vi "Lidar.vi"() -> ()   [LabVIEW 2018]
uses:
  <vilib>/Tufts CEEO ROS for LabVIEW Software/ROS/Code/Console/Servers/ServerSubs/TopicDef.ctl
  <vilib>/Tufts CEEO ROS for LabVIEW Software/ROS/Code/SubVIs/_ROSDirection.ctl
  <vilib>/Utility/inputDevices.llb/keyboardAcquire.vi
  <vilib>/Utility/inputDevices.llb/closeKeyboard.vi
panel:
  out "keyType 3":T1(ring)
  in  "stop 2":bool
  out "new picture":picture
  out "msg out":string
  out "PoseStamped":T2
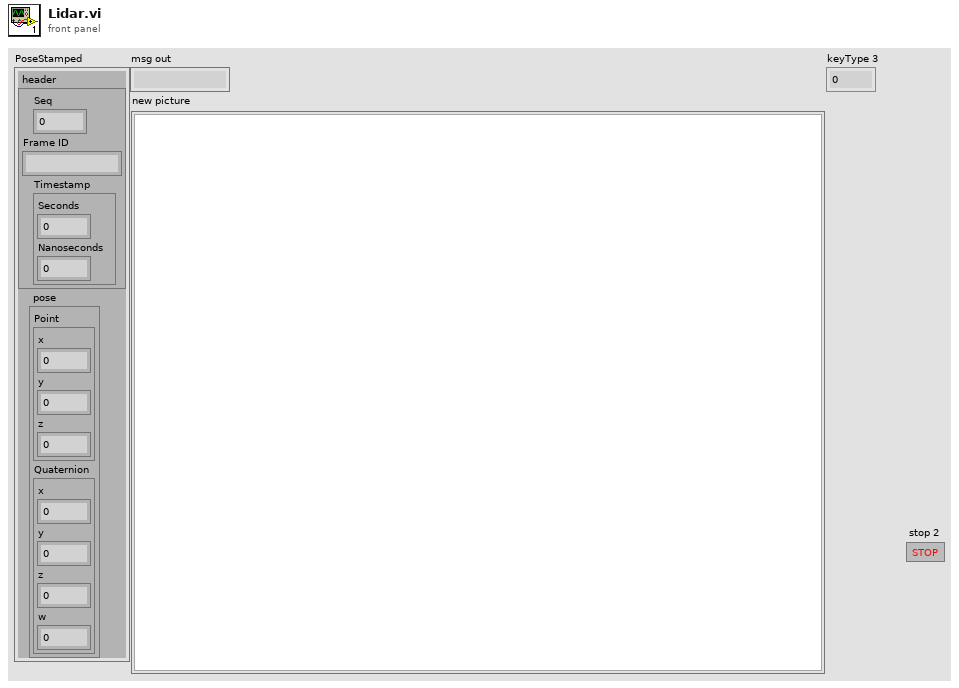
[diagram p1: front panel]
types:
  T1 = enum16{"0", "1", "2", "3", "4", "5", "6", "7", "8", "9", "A", "B", "C", "D", "E", "F", "G", "H", "I", "J", "K", "L", "M", "N", "O", "P", "Q", "R", "S", "T", "U", "V", "W", "X", "Y", "Z", "F1", "F2", "F3", "F4", "F5", "F6", "F7", "F8", "F9", "F10", "F11", "F12", "F13", "F14", "F15", "ADD", "BACK", "BACKSLASH", "CAPITAL", "COMMA", "DECIMAL", "DELETE", "DIVIDE", "DOWN", "END", "EQUALS", "ESCAPE", "GRAVE (`)", "HOME", "INSERT", "LBRACKET", "LCONTROL", "LEFT", "L ALT", "LSHIFT", "LWIN", "MINUS", "MULTIPLY", "NEXT", "NUMLOCK", "NUMPAD_0", "NUMPAD_1", "NUMPAD_2", "NUMPAD_3", "NUMPAD_4", "NUMPAD_5", "NUMPAD_6", "NUMPAD_7", "NUMPAD_8", "NUMPAD_9", "PAUSE", "PERIOD", "PRIOR (PG UP)", "RBRACKET", "RCONTROL", "RETURN", "RIGHT", "R ALT", "RSHIFT", "RWIN", "SCROLL", "SEMICOLON", "SLASH", "SPACE", "SUBTRACT", "TAB", "UP", "ENTER (num pad)", "' (quote)"}
  T2 = cluster{" header":cluster{"Seq":u32, "Frame ID":string, "Timestamp":cluster{"Seconds":i32, "Nanoseconds":i32}}, " pose":cluster{"Point":cluster{"x":dbl, "y":dbl, "z":dbl}, "Quaternion":cluster{"x":dbl, "y":dbl, "z":dbl, "w":dbl}}}
  T3 = typedef "TopicDef.ctl" = cluster{"Topic":string, "Type":string, "Action":T4, "Update (ms)":u16, "queue size":u16}
  T4 = typedef "_ROSDirection.ctl" = enum16{"Node", "Publisher", "Subscriber", "ServiceClient", "ServiceProvider"}
  T5 = typedef "_ROSControl.ctl" = cluster{"topic port":u16, "Node":string, "topic":string, "type":string, "node port":u16, "error ":errorcluster, "Direction":T4, "Update (ms)":u16, "FIFO size":u16}
  T6 = cluster{"Width":u16, "Style":enum32{"Solid", "Dash", "Dot", "DashDot", "DashDotDot"}}
  T7 = cluster{"Linear":cluster{"x":dbl, "y":dbl, "z":dbl}, "Angular":cluster{"x":dbl, "y":dbl, "z":dbl}}
  T8 = enum16{"0", "1", "2", "3", "4", "5", "6", "7", "8", "9", "A", "B", "C", "D", "E", "F", "G", "H", "I", "J", "K", "L", "M", "N", "O", "P", "Q", "R", "S", "T", "U", "V", "W", "X", "Y", "Z", "F1", "F2", "F3", "F4", "F5", "F6", "F7", "F8", "F9", "F10", "F11", "F12", "F13", "F14", "F15", "ADD", "BACK", "BACKSLASH", "CAPITAL", "COMMA", "DECIMAL", "DELETE", "DIVIDE", "DOWN", "END", "EQUALS", "ESCAPE", "GRAVE (`)", "HOME", "INSERT", "LBRACKET", "LCONTROL", "LEFT", "L ALT", "LSHIFT", "LWIN", "MINUS", "MULTIPLY", "NEXT", "NUMLOCK", "NUMPAD_0", "NUMPAD_1", "NUMPAD_2", "NUMPAD_3", "NUMPAD_4", "NUMPAD_5", "NUMPAD_6", "NUMPAD_7", "NUMPAD_8", "NUMPAD_9", "PAUSE", "PERIOD", "PRIOR (PG UP)", "RBRACKET", "RCONTROL", "RETURN", "RIGHT", "R ALT", "RSHIFT", "RWIN", "SCROLL", "SEMICOLON", "SLASH", "SPACE", "SUBTRACT", "TAB", "UP", "ENTER (num pad)", "' (quote)"}[]
  T9 = cluster{"Point":cluster{"x":dbl, "y":dbl, "z":dbl}, "Quaternion":cluster{"x":dbl, "y":dbl, "z":dbl, "w":dbl}}
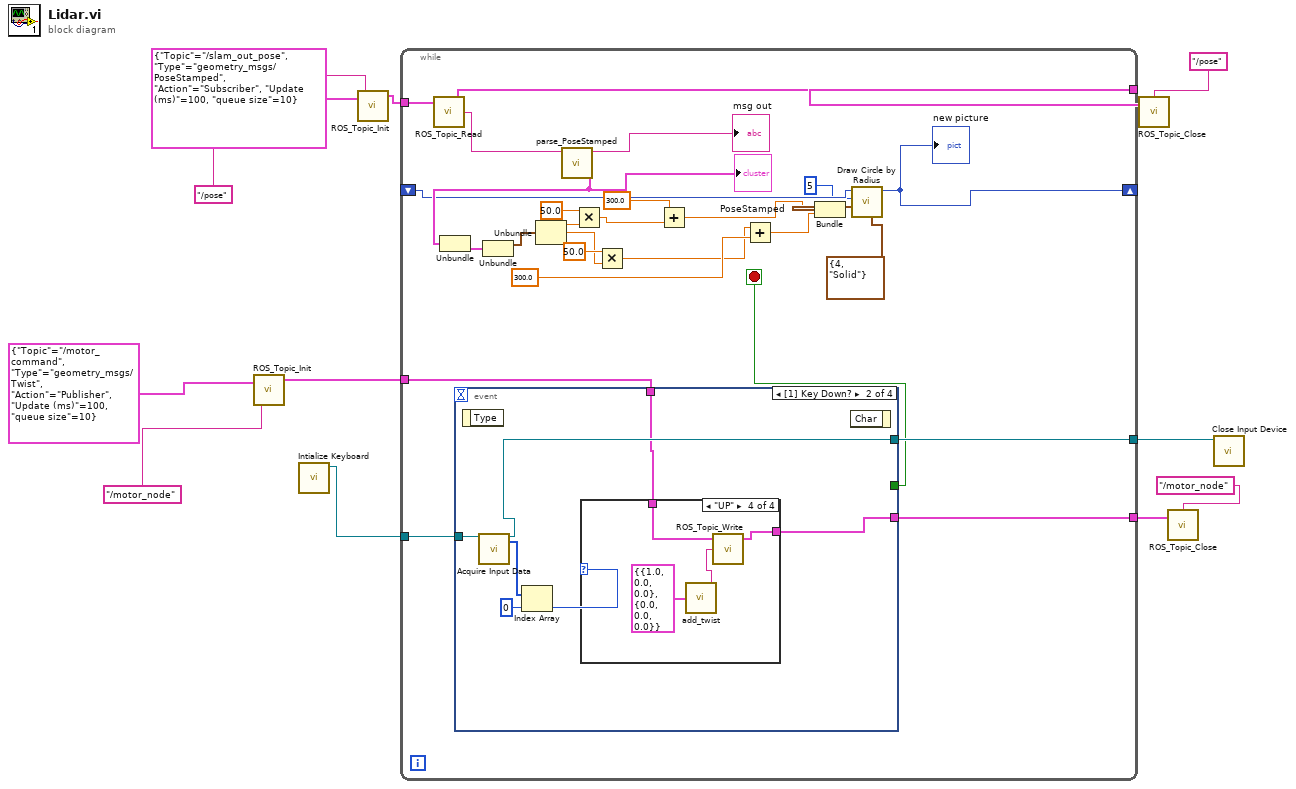
[diagram p0: block diagram]
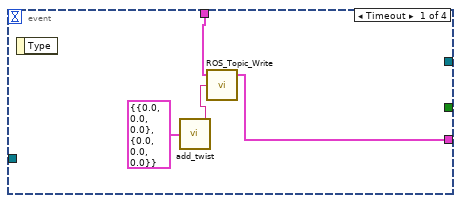
[diagram p2: hidden frame]
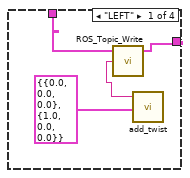
[diagram p3: hidden frame]
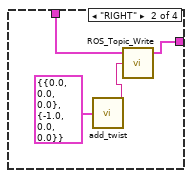
[diagram p4: hidden frame]
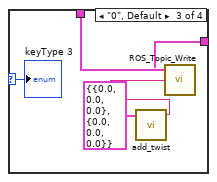
[diagram p5: hidden frame]
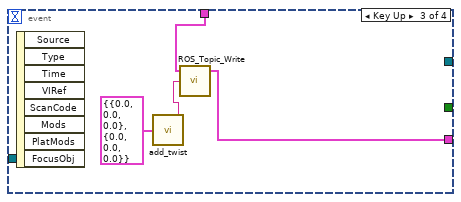
[diagram p6: hidden frame]
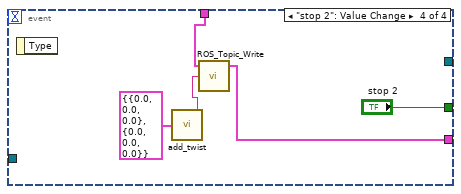
[diagram p7: hidden frame]
diagram:
  n1 = call <vilib>:"ROS_Topic_Init.vi"("Definitions"=T3 {"Topic"="/motor_command", "Type"="geometry_msgs/Twist", "Action"=enum."Publisher", "Update (ms)"=100, "queue size"=10}, "node"="/motor_node") -> ("ROS out"=w3:T5)  [unwired: 1 in, 1 out]
  n2 = call <vilib>:"Intialize Keyboard.vi"() -> ("device ID"=w5:refnum<k1>)  [unwired: 10 in, 1 out]
  n3 = call <vilib>:"ROS_Topic_Init.vi"("Definitions"=T3 {"Topic"="/slam_out_pose", "Type"="geometry_msgs/PoseStamped", "Action"=enum."Subscriber", "Update (ms)"=100, "queue size"=10}, "node"="/pose") -> ("ROS out"=w10:T5)  [unwired: 1 in, 1 out]
  n4 = while {
    tunnel: w10 -> [w39]
    tunnel: [w37] -> w9
    shift-right: [w31] -> _
    shift-left: _ -> [w30]
    tunnel: w5 -> [w17]
    tunnel: [w16] -> w4
    tunnel: w3 -> [w14]
    tunnel: [w13] -> w2
    stop <- w15 stop-if-true
    n5 = call <vilib>:"ROS_Topic_Read.vi"("ROS in"=w39) -> ("Reply"=w38:string, "ROS out"=w37:T5)  [unwired: 2 in, 1 out]
    n6 = event shown="[1] Key Down?" {
      selector: _ -> [_ _ _ _]
      dyn-events: _ -> [_ _ _ _]
      timeout: _ -> [_ _ _ _]
      tunnel: [_ _ _ "stop 2"] -> w15
      tunnel: w17 -> [_ w50 _ _]
      tunnel: [_ w49 _ _] -> w16
      tunnel: w14 -> [w41 w45 w70 w73]
      tunnel: [w42 w44 w68 w74] -> w13
      event Timeout {
        n7 = event-data() -> ()  [unwired: 1 in, 1 out]
        n8 = call <vilib>:"add_twist.vi"("Twist"=T7 {"Linear"={"x"=0.0, "y"=0.0, "z"=0.0}, "Angular"={"x"=0.0, "y"=0.0, "z"=0.0}}) -> ("msg out"=w43:string)  [unwired: 4 in]
        n9 = call <vilib>:"ROS_Topic_Write.vi"("Msg in"=w43, "ROS in"=w41) -> ("ROS out"=w42:T5)  [unwired: 2 in, 1 out]
      }
      event Key Down? {
        n10 = event-data() -> ()  [unwired: 1 in, 1 out]
        n11 = call-poly <vilib>:"Acquire Input Data.vi"("device ID"=w50) -> ("device ID"=w49:refnum<k1>, "keys pressed"=w48:T8)  [unwired: 16 in, 1 out]
        n12 = Index Array(array=w48, index=0) -> (element=w46:T1)
        n13 = case shown="\"UP\"" w46 {
          selector: w46 -> [_ _ w59 _]
          tunnel: w45 -> [w53 w57 w62 w67]
          tunnel: [w52 w56 w61 w65] -> w44
          frame "LEFT" {
            n14 = call <vilib>:"add_twist.vi"("Twist"=T7 {"Linear"={"x"=0.0, "y"=0.0, "z"=0.0}, "Angular"={"x"=1.0, "y"=0.0, "z"=0.0}}) -> ("msg out"=w54:string)  [unwired: 4 in]
            n15 = call <vilib>:"ROS_Topic_Write.vi"("Msg in"=w54, "ROS in"=w53) -> ("ROS out"=w52:T5)  [unwired: 2 in, 1 out]
          }
          frame "RIGHT" {
            n16 = call <vilib>:"add_twist.vi"("Twist"=T7 {"Linear"={"x"=0.0, "y"=0.0, "z"=0.0}, "Angular"={"x"=-1.0, "y"=0.0, "z"=0.0}}) -> ("msg out"=w58:string)  [unwired: 4 in]
            n17 = call <vilib>:"ROS_Topic_Write.vi"("Msg in"=w58, "ROS in"=w57) -> ("ROS out"=w56:T5)  [unwired: 2 in, 1 out]
          }
          frame "0", Default {
            n18 = call <vilib>:"add_twist.vi"("Twist"=T7 {"Linear"={"x"=0.0, "y"=0.0, "z"=0.0}, "Angular"={"x"=0.0, "y"=0.0, "z"=0.0}}) -> ("msg out"=w63:string)  [unwired: 4 in]
            n19 = call <vilib>:"ROS_Topic_Write.vi"("Msg in"=w63, "ROS in"=w62) -> ("ROS out"=w61:T5)  [unwired: 2 in, 1 out]
            "keyType 3" <- w59
          }
          frame "UP" {
            n20 = call <vilib>:"add_twist.vi"("Twist"=T7 {"Linear"={"x"=1.0, "y"=0.0, "z"=0.0}, "Angular"={"x"=0.0, "y"=0.0, "z"=0.0}}) -> ("msg out"=w66:string)  [unwired: 4 in]
            n21 = call <vilib>:"ROS_Topic_Write.vi"("Msg in"=w66, "ROS in"=w67) -> ("ROS out"=w65:T5)  [unwired: 2 in, 1 out]
          }
        }
        n22 = event-data() -> ()  [unwired: 2 in, 1 out]
      }
      event Key Up {
        n23 = event-data() -> ()  [unwired: 1 in, 8 out]
        n24 = call <vilib>:"add_twist.vi"("Twist"=T7 {"Linear"={"x"=0.0, "y"=0.0, "z"=0.0}, "Angular"={"x"=0.0, "y"=0.0, "z"=0.0}}) -> ("msg out"=w71:string)  [unwired: 4 in]
        n25 = call <vilib>:"ROS_Topic_Write.vi"("Msg in"=w71, "ROS in"=w70) -> ("ROS out"=w68:T5)  [unwired: 2 in, 1 out]
      }
      event "stop 2": Value Change {
        n26 = event-data() -> ()  [unwired: 1 in, 1 out]
        n27 = call <vilib>:"add_twist.vi"("Twist"=T7 {"Linear"={"x"=0.0, "y"=0.0, "z"=0.0}, "Angular"={"x"=0.0, "y"=0.0, "z"=0.0}}) -> ("msg out"=w75:string)  [unwired: 4 in]
        n28 = call <vilib>:"ROS_Topic_Write.vi"("Msg in"=w75, "ROS in"=w73) -> ("ROS out"=w74:T5)  [unwired: 2 in, 1 out]
      }
    }
    n29 = call <vilib>:"parse_PoseStamped.vi"("msg in"=w38) -> ("PoseStamped"=w35:T2, "msg out"=→"msg out":string)  [unwired: 8 in, 1 out]
    "PoseStamped" <- w35
    n30 = Unbundle(w35) -> ("pose"=w34:T9)  [unwired: 1 out]
    n31 = Unbundle(w34) -> ("Point"=w33:cluster{"x":dbl, "y":dbl, "z":dbl})  [unwired: 1 out]
    n32 = Unbundle(w33) -> ("x"=w23:dbl, "y"=w19:dbl)  [unwired: 1 out]
    n33 = Multiply(x=50.0, y=w23) -> (x*y=w21:dbl)
    n34 = Multiply(x=50.0, y=w19) -> (x*y=w18:dbl)
    n35 = Add(x=300.0, y=w21) -> (x+y=w26:dbl)
    n36 = Add(x=w18, y=300.0) -> (x+y=w24:dbl)
    n37 = Bundle(w26, w24) -> (w32:cluster{dbl, dbl})  [unwired: 1 in]
    n38 = call <vilib>:"Draw Circle by Radius.vi"("pen"=T6 {"Width"=4, "Style"=enum."Solid"}, "pixel center"=w32, "radius"=i16 5, "picture"=w30) -> ("new picture"=w31:picture)  [unwired: 7 in]
    "new picture" <- w31
  }
  n39 = call <vilib>:"ROS_Topic_Close.vi"("ROS in"=w9, "node"="/pose") -> ()  [unwired: 2 in, 1 out]
  n40 = call <vilib>:"ROS_Topic_Close.vi"("ROS in"=w2, "node"="/motor_node") -> ()  [unwired: 2 in, 1 out]
  n41 = call-poly <vilib>:"Close Input Device.vi"("device ID"=w4) -> ()  [unwired: 9 in, 1 out]
